vi "DataCollectnoTIMELOOPS.vi"() -> ()   [LabVIEW 2009]
uses:
  BaudRateSelector.ctl
  <vilib>/Instr/_visa.llb/Select Event Type.ctl
  <vilib>/Instr/_visa.llb/VISA Configure Serial Port (Instr).vi
  <vilib>/Platform/TimedLoop/scheduler/LVUserAPI/_suppVIs/Create_1kHz_TSource.vi
panel:
  out "Degrees":dbl[](array[numeric]) format="%6.2f"
  in  "LH Calibration File":path
  out "Raw Data":u8[](array[numeric])
  out "Array 2":u32[](array[numeric])
  in  "Sampling Frequency (Hz)":u32 max=120 step=1
  in  "RH COM Port":refnum<visa-resource-name>="COM2"
  in  "LH COM Port":refnum<visa-resource-name>="COM1"
  out "Titles":string[](array[string])
  out "In queue":i32
  out "Interpreted Values":sgl[](array[numeric]) format="%.2f"
  out "Array":u32[](array[numeric])
  in  "stop":bool
  in  "Parity":enum16{"None", "Odd", "Even", "Mark", "Space"}(ring)
  in  "Data Bits":u16=8 min=7 max=8 step=1
  in  "Baud Rate":T1=115200 items=["1200"=1200, "2400"=2400, "4800"=4800, "9600"=9600, "19200"=19200, "38400"=38400, "57600"=57600, "115200"=115200]
  in  "COM Port":refnum<visa-resource-name>="COM3"
  # "Polhemus Serial Information"
  # "If Data Bits = 8, Parity must be \"None\""
  # "0 = As fast as possible"
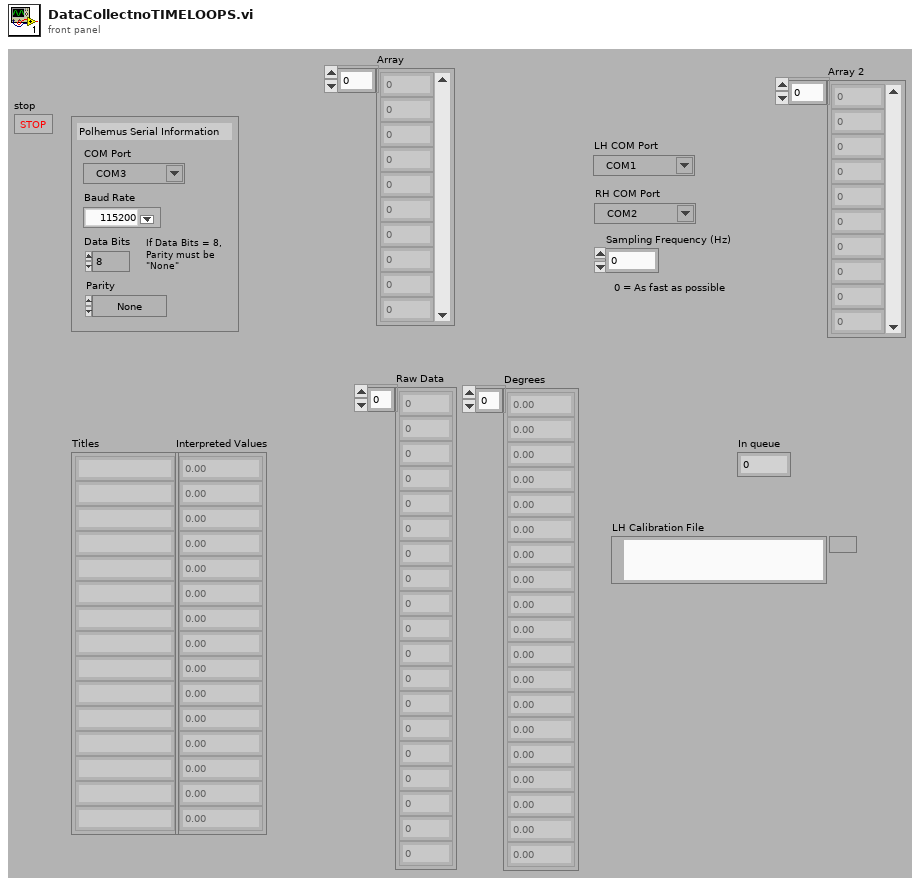
[diagram p1: front panel]
types:
  T1 = typedef "BaudRateSelector.ctl" = u32
  T2 = typedef "Select Event Type.ctl" = u32
  T3 = cluster{"#Bytes":i32[], "Titles":string[], "Format":enum16{"ASCII", "Binary"}, "Units":enum16{"Inches", "Centimeters"}, "Station State":bool[], "#Line Feeds":i32}
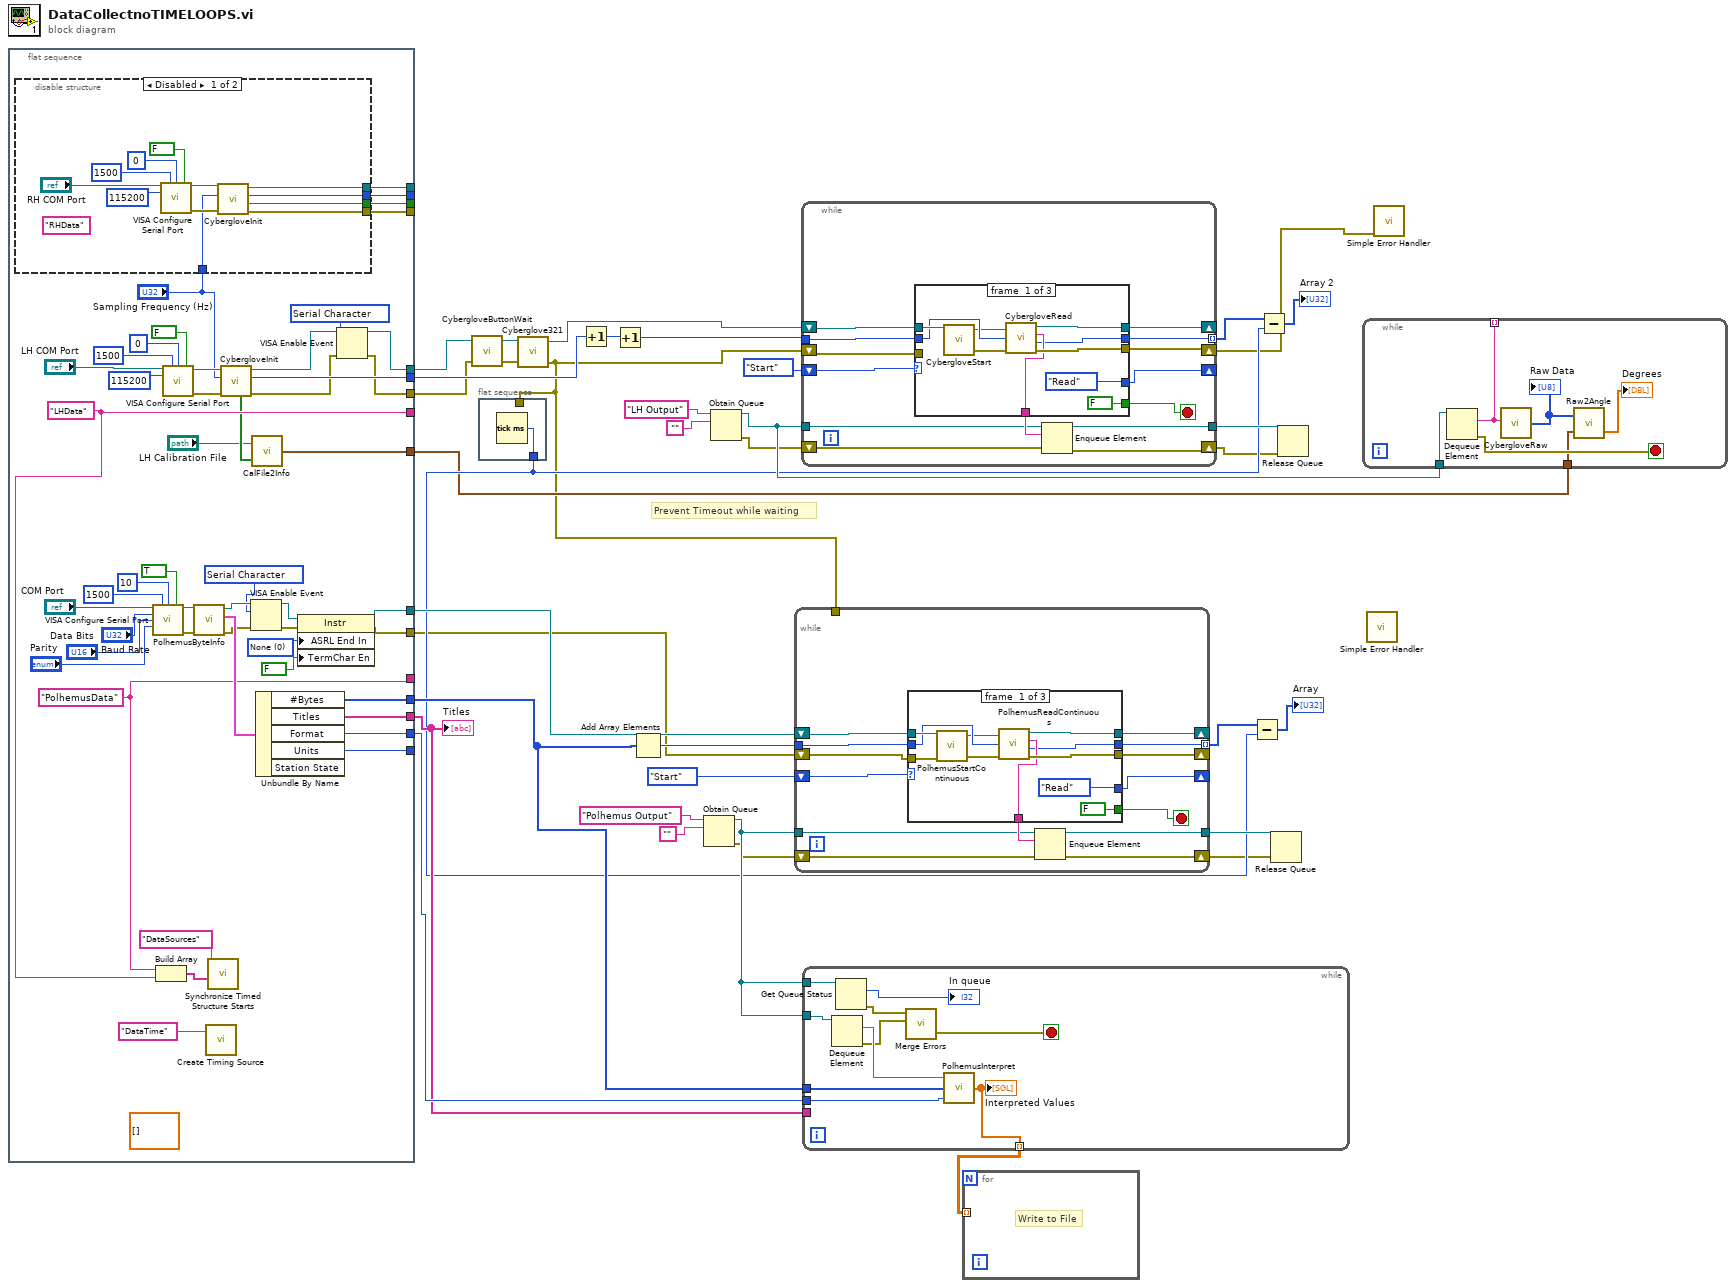
[diagram p0: block diagram]
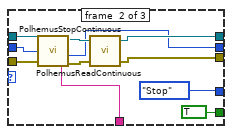
[diagram p2: hidden frame]
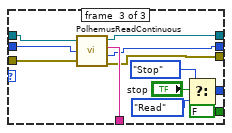
[diagram p3: hidden frame]
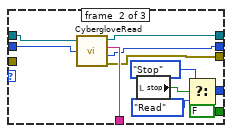
[diagram p4: hidden frame]
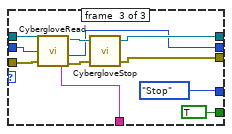
[diagram p5: hidden frame]
diagram:
  # "Prevent Timeout while waiting"
  n1 = flat-sequence {
    tunnel: [w76] -> w36
    tunnel: [w73] -> w3
    tunnel: [w72] -> w30
    tunnel: [w71] -> w25
    tunnel: [w70] -> _
    tunnel: [w69] -> w29
    tunnel: [w62] -> _
    tunnel: [w59] -> _
    tunnel: [w58] -> _
    tunnel: [w57] -> _
    tunnel: [w48] -> w17
    tunnel: [w54] -> w18
    tunnel: [w53] -> _
    tunnel: [w52] -> _
    tunnel: [w47] -> w16
    tunnel: [w38] -> w5
    frame #0 {
      w42 = T2 1073684533 items=["Service Request"=1073684491, "Trigger"=3221168138, "Clear"=1073684493, "VXI Signal"=1073684512, "VXI/VME Interrupt"=3221168161, "VXI/VME Sysfail"=1073684509, "VXI/VME Sysreset"=1073684510, "GPIB CIC"=1073684498, "GPIB Talk"=1073684499, "GPIB Listen"=1073684500, "PXI Interrupt"=1073684514, "Serial Break"=1073684515, "Serial TermChar"=1073684516, "Serial CTS"=1073684521, "Serial DSR"=1073684522, "Serial DCD"=1073684524, "Serial RI"=1073684526, "Serial Character"=1073684533, "USB Interrupt"=1073684535, "All Enabled"=1073709055] ("Event Type")
      w50 = T2 1073684533 items=["Service Request"=1073684491, "Trigger"=3221168138, "Clear"=1073684493, "VXI Signal"=1073684512, "VXI/VME Interrupt"=3221168161, "VXI/VME Sysfail"=1073684509, "VXI/VME Sysreset"=1073684510, "GPIB CIC"=1073684498, "GPIB Talk"=1073684499, "GPIB Listen"=1073684500, "PXI Interrupt"=1073684514, "Serial Break"=1073684515, "Serial TermChar"=1073684516, "Serial CTS"=1073684521, "Serial DSR"=1073684522, "Serial DCD"=1073684524, "Serial RI"=1073684526, "Serial Character"=1073684533, "USB Interrupt"=1073684535, "All Enabled"=1073709055] ("Event Type")
      (unwired) sgl[][] [] ("History Data")
      w59 = "LHData" ("Structure Name")
      w62 = "PolhemusData" ("Structure Name")
      w75 = u16 0 items=["None", "Last Bit", "TermChar"] ("Serial Settings:End Mode for Reads")
      n2 = disable-structure shown="Disabled" {
        disable-tunnel: [w91 _] -> w58
        disable-tunnel: [w90 _] -> w57
        disable-tunnel: [w89 _] -> w53
        disable-tunnel: [w88 _] -> w52
        disable-tunnel: "Sampling Frequency (Hz)" -> [w87 _]
        frame #0 {
          (unwired) "RHData" ("Structure Name")
          n3 = call-poly "VISA Configure Serial Port"("VISA resource name"="RH COM Port", "timeout (10sec)"=u32 1500, "termination char\n(0xA = '\\n' = LF)"=u8 0 ("termination char\n(0xA = '\\n' = LF)"), "Enable Termination\nChar (T)"=FALSE ("Enable Termination\nChar (T)"), "baud rate (9600)"=u32 115200) -> ("VISA resource name out"=w93:refnum<visa-resource-name>, "error out"=w92:errorcluster)  [unwired: 9 in]
          n4 = call "CybergloveInit.vi"("error in (no error)"=w92, "Sampling Frequency (Hz)"=w87, "VISA resource name"=w93) -> ("error out"=w88:errorcluster, "RH?"=w90:bool, "#Sensors"=w91:i32, "VISA resource name out"=w89:refnum<visa-resource-name>)  [unwired: 3 in, 2 out]
        }
        frame #1 {
        }
      }
      n5 = call-poly "VISA Configure Serial Port"("VISA resource name"="COM Port", "timeout (10sec)"=u32 1500, "termination char\n(0xA = '\\n' = LF)"=u8 10 ("termination char\n(0xA = '\\n' = LF)"), "Enable Termination\nChar (T)"=TRUE ("Enable Termination\nChar (T)"), "baud rate (9600)"="Baud Rate", "data bits (8)"="Data Bits", "parity (0:none)"="Parity") -> ("VISA resource name out"=w81:refnum<visa-resource-name>, "error out"=w80:errorcluster)  [unwired: 7 in]
      n6 = Build Array(w62, w59) -> (w61:string[])
      n7 = call-poly "VISA Configure Serial Port"("VISA resource name"="LH COM Port", "timeout (10sec)"=u32 1500, "termination char\n(0xA = '\\n' = LF)"=u8 0 ("termination char\n(0xA = '\\n' = LF)"), "Enable Termination\nChar (T)"=FALSE ("Enable Termination\nChar (T)"), "baud rate (9600)"=u32 115200) -> ("VISA resource name out"=w56:refnum<visa-resource-name>, "error out"=w55:errorcluster)  [unwired: 9 in]
      n8 = call "PolhemusByteInfo.vi"("error in (no error)"=w80, "VISA resource name"=w81) -> ("error out"=w46:errorcluster, "Polhemus Info"=w77:T3, "VISA resource name out"=w44:refnum<visa-resource-name>)  [unwired: 5 in]
      n9 = call-poly <vilib>:"Create Timing Source.vi"("name (in)"="DataTime") -> ()  [unwired: 9 in, 2 out]
      n10 = call <vilib>:"Synchronize Timed Structure Starts.vi"("timed structure names"=w61, "synchronization group name"="DataSources") -> ()  [unwired: 8 in, 2 out]
      n11 = call "CybergloveInit.vi"("error in (no error)"=w55, "Sampling Frequency (Hz)"="Sampling Frequency (Hz)", "VISA resource name"=w56) -> ("error out"=w49:errorcluster, "#Sensors"=w54:i32, "VISA resource name out"=w51:refnum<visa-resource-name>, "Sensors Active"=w40:bool[])  [unwired: 3 in, 2 out]
      n12 = VISA Enable Event(8:w46, 10:w42, 11:w44) -> (0:w45:errorcluster, 3:w43:refnum<visa-resource-name>)  [unwired: 1 in]
      n13 = call "CalFile2Info.vi"("file (use dialog)"="LH Calibration File", "Sensors Active"=w40) -> ("Array"=w38:cluster{"Offset":dbl, "Gain":dbl}[])  [unwired: 2 in]
      n14 = Unbundle By Name(w77) -> ("#Bytes"=w72:i32[], "Titles"=w71:string[], "Format"=w69:enum16{"ASCII", "Binary"}, "Units"=w70:enum16{"Inches", "Centimeters"})  [unwired: 1 out]
      n15 = property class="Instr"(reference=w43, error in=w45, "ASRL End In"=w75, "TermChar En"=FALSE ("Message Based Settings:Termination Character Enable")) -> (reference out=w76:refnum<visa-resource-name>, error out=w73:errorcluster)
      n16 = VISA Enable Event(8:w49, 10:w50, 11:w51) -> (0:w47:errorcluster, 3:w48:refnum<visa-resource-name>)  [unwired: 1 in]
    }
  }
  n17 = call "CybergloveButtonWait.vi"("error in (no error)"=w16, "VISA resource name"=w17) -> ("error out"=w14:errorcluster, "VISA resource name out"=w15:refnum<visa-resource-name>)  [unwired: 2 in]
  n18 = flat-sequence {
    tunnel: w1 -> [_]
    tunnel: [w99] -> w10
    frame #0 {
      n19 = Tick Count (ms)() -> (millisecond timer value=w99:u32)
    }
  }
  n20 = call "Cyberglove321.vi"("error in (no error)"=w14, "VISA resource name"=w15) -> ("error out"=w1:errorcluster, "VISA resource name out"=w2:refnum<visa-resource-name>)  [unwired: 2 in]
  n21 = Increment(x=w18) -> (x+1=w12:i32)
  n22 = Increment(x=w12) -> (x+1=w11:i32)
  n23 = Add Array Elements(numeric array=w30) -> (sum=w37:i32)
  n24 = Obtain Queue(name (unnamed)="Polhemus Output", element data type="") -> (queue out=w27:refnum<queue>, error out=w9:errorcluster)  [unwired: 3 in, 1 out]
  n25 = Obtain Queue(name (unnamed)="LH Output", element data type="") -> (queue out=w13:refnum<queue>, error out=w7:errorcluster)  [unwired: 3 in, 1 out]
  n26 = while {
    tunnel: w37 -> [w112]
    shift-right: [w109] -> _
    shift-left: enum16{"Start", "Read", "Stop"}."Start" -> [w111]
    shift-right: [w110] -> _
    shift-left: w36 -> [w113]
    tunnel: [w107] -> w34 mode=indexing
    tunnel: w27 -> [w105]
    tunnel: [w104] -> w28
    tunnel: w1 -> [_]
    shift-right: [w102] -> w8
    shift-left: w9 -> [w103]
    shift-right: [w100] -> _
    shift-left: w3 -> [w101]
    stop <- w108 stop-if-true
    n27 = case shown="\"Read\"" w111 {
      tunnel: w113 -> [w124 w131 w147]
      tunnel: [w117 w134 w146] -> w106
      tunnel: w112 -> [w122 w135 w145]
      tunnel: w101 -> [w123 w130 w138]
      tunnel: [w119 w127 w139] -> w110
      tunnel: [w118 w126 w137] -> w100
      tunnel: [enum16{"Start", "Read", "Stop"}."Read" enum16{"Start", "Read", "Stop"}."Stop" w141] -> w109
      tunnel: [FALSE TRUE FALSE] -> w108
      tunnel: [w114 w125 w136] -> w107
      frame #0 {
        n28 = call "PolhemusStartContinuous.vi"("error in (no error)"=w123, "VISA resource name"=w124) -> ("error out"=w120:errorcluster, "VISA resource name out"=w121:refnum<visa-resource-name>)  [unwired: 2 in]
        n29 = call "PolhemusReadContinuous.vi"("VISA resource name"=w121, "Byte Sum"=w122, "error in (no error)"=w120) -> ("VISA resource name out"=w119:refnum<visa-resource-name>, "Polhemus Output"=w117:string, "Time"=w114:u32, "error out"=w118:errorcluster)
      }
      frame #1 {
        n30 = call "PolhemusReadContinuous.vi"("VISA resource name"=w131, "Byte Sum"=w135, "error in (no error)"=w130) -> ("VISA resource name out"=w129:refnum<visa-resource-name>, "Polhemus Output"=w134:string, "Time"=w125:u32, "error out"=w128:errorcluster)
        n31 = call "PolhemusStopContinuous.vi"("error in (no error)"=w128, "VISA resource name"=w129) -> ("error out"=w126:errorcluster, "VISA resource name out"=w127:refnum<visa-resource-name>)  [unwired: 2 in]
      }
      frame #2 {
        n32 = call "PolhemusReadContinuous.vi"("VISA resource name"=w147, "Byte Sum"=w145, "error in (no error)"=w138) -> ("VISA resource name out"=w139:refnum<visa-resource-name>, "Polhemus Output"=w146:string, "Time"=w136:u32, "error out"=w137:errorcluster)
        n33 = Select(t=enum16{"Start", "Read", "Stop"}."Stop", s="stop", f=enum16{"Start", "Read", "Stop"}."Read") -> (s? t:f=w141:enum16{"Start", "Read", "Stop"})
      }
    }
    n34 = Enqueue Element(queue=w105, element=w106, error in (no error)=w103) -> (queue out=w104:refnum<queue>, error out=w102:errorcluster)  [unwired: 1 in, 1 out]
  }
  n35 = while {
    tunnel: w11 -> [w160]
    shift-right: [w157] -> _
    shift-left: enum16{"Start", "Read", "Stop"}."Start" -> [w159]
    shift-right: [w158] -> _
    shift-left: w2 -> [w161]
    tunnel: [w155] -> w23 mode=indexing
    tunnel: w13 -> [w153]
    tunnel: [w152] -> w19
    shift-right: [w150] -> w6
    shift-left: w7 -> [w151]
    shift-right: [w148] -> w4
    shift-left: w1 -> [w149]
    stop <- w156 stop-if-true
    n36 = case shown="\"Stop\"" w159 {
      tunnel: w161 -> [w171 w182 w189]
      tunnel: [w165 w181 w192] -> w154
      tunnel: w160 -> [w170 w180 w193]
      tunnel: [w167 w175 w186] -> w158
      tunnel: [w166 w174 w185] -> w148
      tunnel: [enum16{"Start", "Read", "Stop"}."Read" w177 enum16{"Start", "Read", "Stop"}."Stop"] -> w157
      tunnel: [FALSE FALSE TRUE] -> w156
      tunnel: [w162 w173 w184] -> w155
      tunnel: w149 -> [_ _ w183]
      frame #0 {
        n37 = call "CybergloveStart.vi"("VISA resource name"=w171) -> ("error out"=w168:errorcluster, "VISA resource name out"=w169:refnum<visa-resource-name>)  [unwired: 3 in]
        n38 = call "CybergloveRead.vi"("VISA resource name"=w169, "Bytes"=w170, "error in (no error)"=w168) -> ("VISA resource name out"=w167:refnum<visa-resource-name>, "Cyberglove Output"=w165:string, "Time"=w162:u32, "error out"=w166:errorcluster)
      }
      frame #1 {
        n39 = call "CybergloveRead.vi"("VISA resource name"=w182, "Bytes"=w180) -> ("VISA resource name out"=w175:refnum<visa-resource-name>, "Cyberglove Output"=w181:string, "Time"=w173:u32, "error out"=w174:errorcluster)  [unwired: 1 in]
        n40 = local read "stop"() -> (w172:bool)
        n41 = Select(t=enum16{"Start", "Read", "Stop"}."Stop", s=w172, f=enum16{"Start", "Read", "Stop"}."Read") -> (s? t:f=w177:enum16{"Start", "Read", "Stop"})
      }
      frame #2 {
        n42 = call "CybergloveRead.vi"("VISA resource name"=w189, "Bytes"=w193, "error in (no error)"=w183) -> ("VISA resource name out"=w188:refnum<visa-resource-name>, "Cyberglove Output"=w192:string, "Time"=w184:u32, "error out"=w187:errorcluster)
        n43 = call "CybergloveStop.vi"("error in (no error)"=w187, "VISA resource name"=w188) -> ("error out"=w185:errorcluster, "VISA resource name out"=w186:refnum<visa-resource-name>)  [unwired: 2 in]
      }
    }
    n44 = Enqueue Element(queue=w153, element=w154, error in (no error)=w151) -> (queue out=w152:refnum<queue>, error out=w150:errorcluster)  [unwired: 1 in, 1 out]
  }
  n45 = while {
    tunnel: w27 -> [w203]
    tunnel: w30 -> [w201]
    tunnel: w29 -> [w200]
    tunnel: w27 -> [w199]
    tunnel: [w194] -> w26 mode=indexing
    tunnel: w25 -> [_]
    stop <- w197 stop-if-true
    n46 = Dequeue Element(queue=w203) -> (element=w202:string, error out=w196:errorcluster)  [unwired: 2 in, 2 out]
    n47 = Get Queue Status(queue=w199) -> (# pending remove=→"In queue":i32, error out=w195:errorcluster)  [unwired: 2 in, 6 out]
    n48 = call <vilib>:"Merge Errors.vi"("error in 2 (no error)"=w196, "error in 1 (no error)"=w195) -> ("error out"=w197:errorcluster)  [unwired: 5 in]
    n49 = call "PolhemusInterpret.vi"("Format"=w200, "#Bytes"=w201, "Polhemus Output"=w202) -> ("Interpreted Values"=w194:sgl[])  [unwired: 1 in]
    "Interpreted Values" <- w194
  }
  n50 = for {
    tunnel: w26 -> [_] mode=indexing
    # "Write to File"
  }
  n51 = Subtract(x=w34, y=w10) -> (x-y=→"Array":u32[])
  n52 = Subtract(x=w23, y=w10) -> (x-y=→"Array 2":u32[])
  n53 = Release Queue(queue=w28, error in (no error)=w8) -> ()  [unwired: 1 in, 3 out]
  n54 = Release Queue(queue=w19, error in (no error)=w6) -> ()  [unwired: 1 in, 3 out]
  n55 = while {
    tunnel: w13 -> [w209]
    tunnel: [w207] -> _ mode=indexing
    tunnel: w5 -> [w206]
    stop <- w208 stop-if-true
    n56 = Dequeue Element(queue=w209) -> (element=w207:string, error out=w208:errorcluster)  [unwired: 2 in, 2 out]
    n57 = call "CybergloveRaw.vi"("Cyberglove Out"=w207) -> ("Raw Data"=w205:u8[])
    "Raw Data" <- w205
    n58 = call "Raw2Angle.vi"("Calibration"=w206, "Raw Data"=w205) -> ("Degrees"=→"Degrees":dbl[])  [unwired: 1 out]
  }
  n59 = call <vilib>:"Simple Error Handler.vi"() -> ()  [unwired: 5 in, 5 out]
  n60 = call <vilib>:"Simple Error Handler.vi"("error in (no error)"=w4) -> ()  [unwired: 4 in, 5 out]
  "Titles" <- w25
